vi "test_distributeVerticalCentersShouldDoNothing.vi"(11 "Test Case In":refnum<class "DistributeCentersTests.lvclass">) -> (0 "error out":errorcluster, 3 "Test Case Out":refnum<class "DistributeCentersTests.lvclass">)   [LabVIEW 2023, in "DistributeCentersTests.lvclass"]
uses:
  DistributeCentersTests.lvclass
  source/Ctrls/alignment.ctl
  <vilib>/Astemes/LUnit/Test Case.lvclass/Test Case.ctl
  source/Misc/getBoundsRect.vi
  <vilib>/Astemes/LUnit/Core/LUnit Test Case/Private/Append Fail Result.vi
  <vilib>/Astemes/LUnit/Core/LUnit Test Case/Private/Append Pass Result.vi
  source/Misc/processUseControlBodyOnlyFlag_start.vi
  source/Misc/processUseControlBodyOnlyFlag_end.vi
  <vilib>/Astemes/LUnit/Core/LUnit Test Case/Private/Run In UI.vi
  <vilib>/Utility/error.llb/Clear Errors.vi
  source/Misc/hideCaption&Label.vi
  source/Misc/setCaption&LabelVisibility.vi
  DistributeCentersTests.lvclass/DistributeCentersTests.ctl
  <vilib>/Astemes/LUnit/Test Case.lvclass
panel:
  in  "Numeric_bottommost":dbl
  in  "firstItem_topmost":string
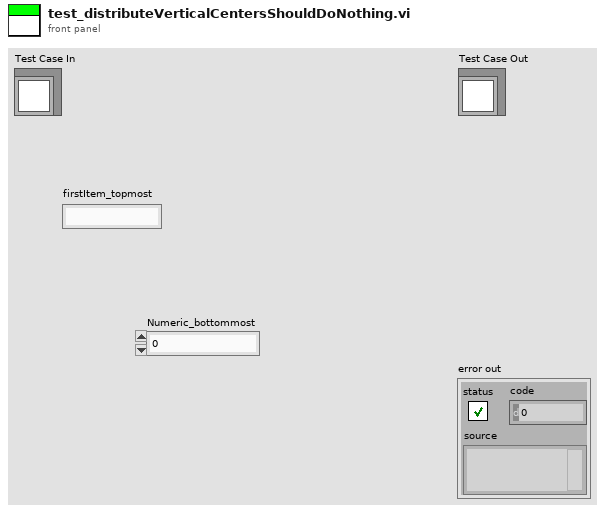
[diagram p1: front panel]
types:
  T1 = typedef "alignment.ctl" = enum16{"None", "AlignTop", "AlignBottom", "AlignHorizontalCenters", "AlignLeft", "AlignRight", "AlignVerticalCenters"}
  T2 = typedef "LVPositionTypeDef.ctl" = cluster{"Left":i32, "Top":i32}
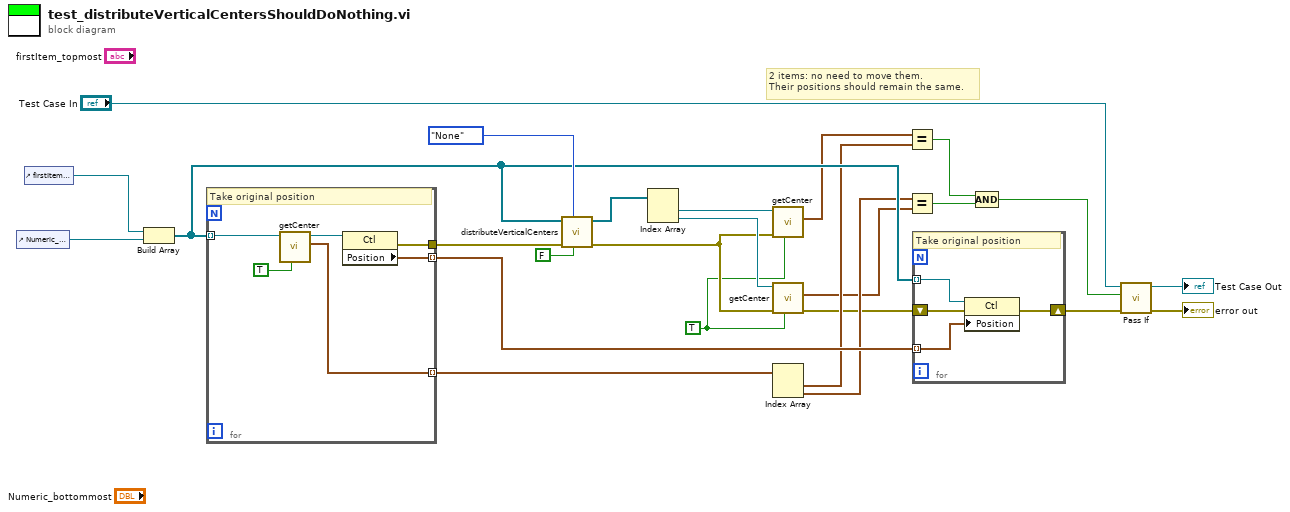
[diagram p0: block diagram]
diagram:
  w3 = TRUE ("useControlBodyOnly")
  # "2 items: no need to move them.\nTheir positions should remain the same."
  n1 = control-ref of="Numeric_bottommost"() -> (w18:refnum<vi>)
  n2 = control-ref of="firstItem_topmost"() -> (w19:refnum<vi>)
  n3 = Build Array(w19, w18) -> (w17:refnum<vi>[])
  n4 = for {
    tunnel: w17 -> [w31] mode=indexing
    tunnel: [w30] -> w15 mode=indexing
    tunnel: [w29] -> w22
    tunnel: [w27] -> w11 mode=indexing
    # "Take original position"
    n5 = call "getCenter.vi"("useControlBodyOnly"=TRUE, "ref"=w31) -> ("center"=w27:cluster{"horizontal":i32, "vertical":i32}, "ref(dup)"=w28:refnum<vi>)  [unwired: 7 in, 1 out]
    n6 = property class="Ctl"(reference=w28) -> (error out=w29:errorcluster, "Position"=w30:T2)  [unwired: 1 in, 1 out]
  }
  n7 = call "distributeVerticalCenters.vi"("useControlBodyOnly"=FALSE, "horizontalAlignment"=alignment."None" ("verticalAlignment"), "error in (no error)"=w22, "refs"=w17) -> ("error out"=w4:errorcluster, "refs(dup)"=w16:refnum<vi>[])  [unwired: 6 in]
  n8 = Index Array(array=w16) -> (element #1=w12:refnum<vi>, element #2=w5:refnum<vi>)  [unwired: 2 in]
  n9 = call "getCenter.vi"("useControlBodyOnly"=w3, "error in (no error)"=w4, "ref"=w12) -> ("center"=w10:cluster{"horizontal":i32, "vertical":i32})  [unwired: 6 in, 2 out]
  n10 = call "getCenter.vi"("useControlBodyOnly"=w3, "error in (no error)"=w4, "ref"=w5) -> ("error out"=w2:errorcluster, "center"=w1:cluster{"horizontal":i32, "vertical":i32})  [unwired: 6 in, 1 out]
  n11 = Index Array(array=w11) -> (element #1=w14:cluster{"horizontal":i32, "vertical":i32}, element #2=w13:cluster{"horizontal":i32, "vertical":i32})  [unwired: 2 in]
  n12 = Equal?(x=w10, y=w14) -> (x = y?=w9:bool)
  n13 = Equal?(x=w13, y=w1) -> (x = y?=w8:bool)
  n14 = for {
    tunnel: w17 -> [w35] mode=indexing
    tunnel: w15 -> [w34] mode=indexing
    shift-right: [w33] -> w6
    shift-left: w2 -> [w32]
    # "Take original position"
    n15 = property class="Ctl"(reference=w35, error in=w32, "Position"=w34) -> (error out=w33:errorcluster)  [unwired: 1 out]
  }
  n16 = Compound Arithmetic op=AND(w9, w8) -> (w7:bool)
  n17 = call <vilib>:"Pass If.vi"("error in (no error)"=w6, "Pass?"=w7, "LUnit Test Case In"="Test Case In") -> ("error out"=→"error out":errorcluster, "LUnit Test Case Out"=→"Test Case Out":refnum<class "DistributeCentersTests.lvclass">)  [unwired: 7 in]
